vi "HMP4040 Close_v2.vi"(8 "error in (no error)":errorcluster, 11 "HMP VISA":refnum<visa-resource-name>="HMP4040_FTS2") -> (0 "error out":errorcluster)   [LabVIEW 2022 SP3]
doc: "This VI will close the HMP Power Supply VISA session"
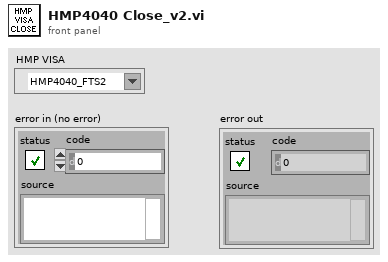
[diagram p1: front panel]
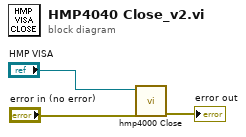
[diagram p0: block diagram]
diagram:
  n1 = call "hmp4000 Close.vi"("error in (no error)"="error in (no error)", "VISA resource name"="HMP VISA") -> ("error out"=→"error out":errorcluster)  [unwired: 9 in]
